vi "Coerce AO.vi"(8 "error in (no error)":errorcluster, 11 "Instrument.Lockin":refnum<class "Instrument.Lockin.lvclass">) -> (0 "error out":errorcluster, 3 "Instrument.Lockin out":refnum<class "Instrument.Lockin.lvclass">)   [LabVIEW 2016, in "Instrument.Lockin.lvclass"]
uses:
  Instrument.Lockin.lvclass
  Instrument.Lockin.lvclass/Instrument.Lockin.ctl
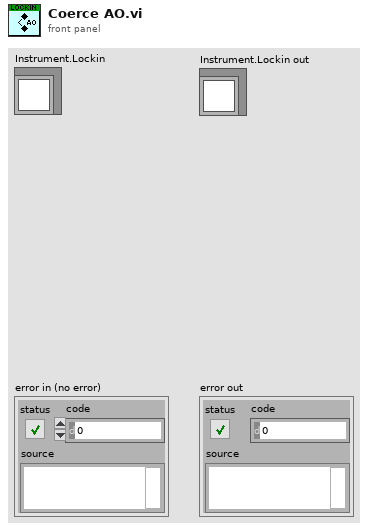
[diagram p1: front panel]
types:
  T1 = typedef "Lockin.DAQ.lvclass/AO.config-array.ctl" = T2[]
  T2 = typedef "Lockin.DAQ.lvclass/AO.config-cluster.ctl" = cluster{"AO.channels":tag, "AO.Range":T3, "output terminal configuration":i32, "DAQ Type":T4}
  T3 = typedef "Lockin.DAQ.lvclass/446xAO-enum.ctl" = enum16{"±0.1 V", "±1.0 V", "±10.0 V"}
  T4 = typedef "Lockin.DAQ.lvclass/DAQType-enum.ctl" = enum16{"None", "USB 4431", "PXI 446x"}
  T5 = typedef "Lockin.DAQ.lvclass/AO-cluster.ctl" = cluster{"Ch":i32[], "Amp (V)":dbl[], "DC (V)":dbl[], "f (Hz)":dbl[], "Phase (°)":dbl[], "Function":T6[], "Sweep?":bool[]}
  T6 = typedef "Lockin.DAQ.lvclass/Function-enum.ctl" = enum16{"Sine", "Triangle", "Square", "Sawtooth"}
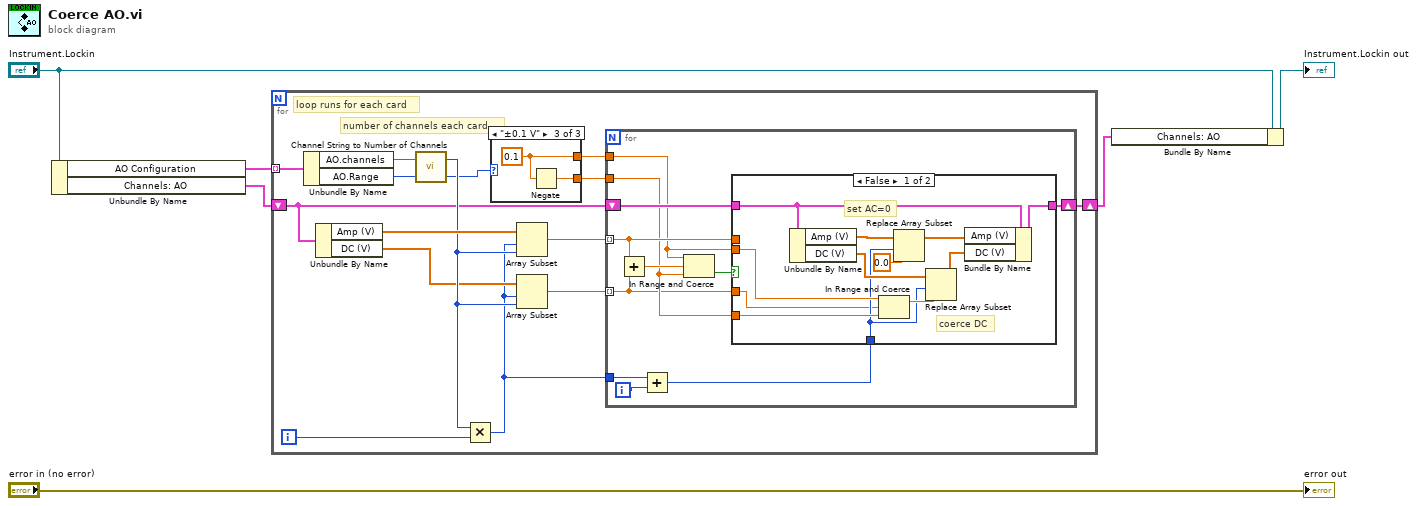
[diagram p0: block diagram]
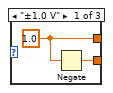
[diagram p2: hidden frame]
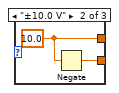
[diagram p3: hidden frame]
diagram:
  n1 = Unbundle By Name("Instrument.Lockin") -> ("AO Configuration"=w6:T1, "Channels: AO"=w4:T5)
  n2 = for {
    tunnel: w6 -> [w20] mode=indexing
    shift-right: [w11] -> w2
    shift-left: w4 -> [w12]
    i -> [w18]
    # "number of channels each card"
    # "loop runs for each card"
    n3 = Unbundle By Name(w20) -> ("AO.channels"=w19:tag, "AO.Range"=w9:T3)
    n4 = Unbundle By Name(w12) -> ("Amp (V)"=w17:dbl[], "DC (V)"=w15:dbl[])
    n5 = call "Channel String to Number of Channels.vi"("Channels String"=w19) -> ("# channels"=w16:i32)  [unwired: 2 in]
    n6 = Multiply(x=w16, y=w18) -> (x*y=w10:i32)
    n7 = case shown="\"±0.1 V\"" w9 {
      tunnel: [w22 w24 w26] -> w7
      tunnel: [w21 w23 w25] -> w8
      frame "±1.0 V" {
        w22 = 1.0
        n8 = Negate(x=w22) -> (-x=w21:dbl)
      }
      frame "±10.0 V" {
        w24 = 10.0
        n9 = Negate(x=w24) -> (-x=w23:dbl)
      }
      frame "±0.1 V" {
        w26 = 0.1
        n10 = Negate(x=w26) -> (-x=w25:dbl)
      }
    }
    n11 = Array Subset(array=w17, index=w10, length=w16) -> (w13:dbl[])
    n12 = Array Subset(array=w15, index=w10, length=w16) -> (w14:dbl[])
    n13 = for {
      tunnel: w7 -> [w29]
      tunnel: w8 -> [w28]
      tunnel: w14 -> [w27] mode=indexing
      tunnel: w13 -> [w35] mode=indexing
      tunnel: w10 -> [w31]
      shift-right: [w33] -> w11
      shift-left: w12 -> [w34]
      i -> [w32]
      n14 = Add(x=w35, y=w27) -> (x+y=w37:dbl)
      n15 = Add(x=w31, y=w32) -> (x+y=w30:i32)
      n16 = In Range and Coerce(upper limit=w29, x=w37, lower limit=w28) -> (In Range?=w36:bool)  [unwired: 1 out]
      n17 = case shown="False" w36 {
        tunnel: w35 -> [_ _]
        tunnel: w34 -> [w49 w50]
        tunnel: [w48 w50] -> w33
        tunnel: w30 -> [w39 _]
        tunnel: w29 -> [w41 _]
        tunnel: w28 -> [w40 _]
        tunnel: w27 -> [w38 _]
        frame False {
          # "set AC=0"
          # "coerce DC"
          n18 = Unbundle By Name(w49) -> ("Amp (V)"=w47:dbl[], "DC (V)"=w45:dbl[])
          n19 = In Range and Coerce(upper limit=w41, x=w38, lower limit=w40) -> (coerced(x)=w42:dbl)  [unwired: 1 out]
          n20 = Replace Array Subset(array=w47, new element=0.0 ("new element/subarray"), index=w39) -> (w46:dbl[])
          n21 = Replace Array Subset(array=w45, new element=w42, index=w39) -> (w44:dbl[])
          n22 = Bundle By Name(cluster=w49, "Amp (V)"=w46, "DC (V)"=w44) -> (w48:T5)
        }
        frame True {
        }
      }
    }
  }
  n23 = Bundle By Name(cluster="Instrument.Lockin", "Channels: AO"=w2) -> (→"Instrument.Lockin out":refnum<class "Instrument.Lockin.lvclass">)
  "error out" <- "error in (no error)"
